vi "PH_TKTDS-30xx.PC Set Channel Position.vi"(0 "i ref in":refnum<vi>, 2 "Channel Name":string(combo)="CH1", 3 "Position (0)":dbl, 5 "error IO":errorcluster) -> (14 "i ref out":refnum<vi>, 19 "error out":errorcluster)   [LabVIEW 2014, in "PH_TKTDS-30xx.lvlib"]
doc: "This case sets the position of the specified channel at the display in display divisions."
uses:
  PH_TKTDS-30xx.lvlib
  instr.lib/TKDS3032-PHELIX/tktds3032-PHELIX - Driver np.lvlib
  PH_Basics/PH_Common/PH_Common.lvlib
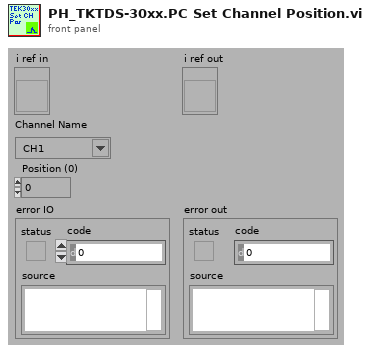
[diagram p1: front panel]
types:
  T1 = typedef "PH_TKTDS-30xx.lvlib/PH_TKTDS-30xx.i attribute.ctl" = cluster{"Default VISA Resource":string, "VISA Resource Name":refnum<visa-resource-name>, "Revision":cluster{"Instrument Driver":string, "Instrument Firmware":string}, "Selftest":cluster{"Result":u32, "Message":string}, "Channels":T2[], "Trigger Configuration":T3, "Acquisition Configuration":T4, "Fetched Waveforms":T5[], "GUI Refs":T6, "GUI Refs Channels":refnum<vi>[], "State":T7, "Error Message":string, "Allow Prdc Loop?":bool}
  T2 = typedef "PH_TKTDS-30xx.lvlib/PH_TKTDS-30xx.Channel Config.ctl" = cluster{"Channel Name":string, "Input Impedance":string, "Max Input Frequency":string, "Vertical Coupling":i32, "Channel Enabled":bool, "Probe Attenuation":dbl, "Vertical Range":dbl, "Vertical Offset":dbl}
  T3 = typedef "PH_TKTDS-30xx.lvlib/PH_TKTDS-30xx.Trigger Config.ctl" = cluster{"Source":string, "Slope":i32, "Level [V]":dbl}
  T4 = typedef "PH_TKTDS-30xx.lvlib/PH_TKTDS-30xx.Acquisition Config.ctl" = cluster{"Time base":dbl, "Record Length":u16, "Start Time":dbl, "Type":i32, "Continuous":bool}
  T5 = typedef "PH_TKTDS-30xx.lvlib/PH_TKTDS-30xx.fetched Waveform.ctl" = cluster{"Source":string, "Actual Points":u32, "Initial X":dbl, "X Increment":dbl, "Waveform Array":dbl[]}
  T6 = typedef "PH_TKTDS-30xx.lvlib/PH_TKTDS-30xx.GUI Refs.ctl" = cluster{"Trigger":refnum<vi>, "Acquisition":refnum<vi>, "Graph":refnum<vi>, "State":refnum<vi>, "Delete":refnum<vi>, "Channel to be positioned":refnum<vi>, "Postion":refnum<vi>, "Display Intensity":refnum<vi>, "VISA Resource":refnum<vi>}
  T7 = typedef "PH_StatusHandler.lvlib/PH_StatusHandler.Status.ctl" = i16
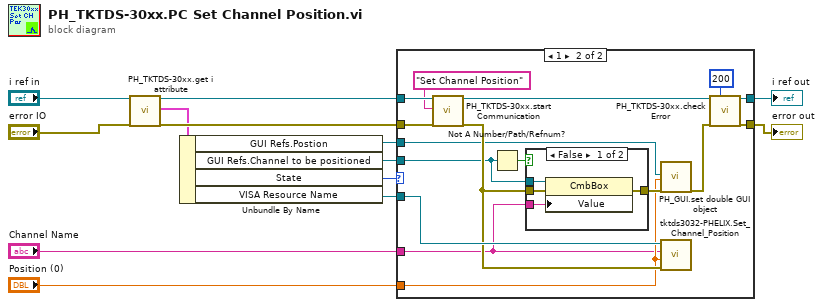
[diagram p0: block diagram]
diagram:
  n1 = call "PH_TKTDS-30xx.get i attribute.vi"("i ref in"="i ref in", "error in (no error)"="error IO") -> ("i ref out"=w8:refnum<vi>, "i attribute"=w10:T1, "error out"=w12:errorcluster)  [unwired: 15 in]
  n2 = Unbundle By Name(w10) -> ("GUI Refs.Postion"=w2:refnum<vi>, "GUI Refs.Channel to be positioned"=w3:refnum<vi>, "State"=w1:T7, "VISA Resource Name"=w11:refnum<visa-resource-name>)
  n3 = case shown="1" w1 {
    tunnel: w8 -> [w15 w31]
    tunnel: w11 -> [_ w30]
    tunnel: [w14 w29] -> w6
    tunnel: w12 -> [w14 w24]
    tunnel: [w15 w28] -> w13
    tunnel: "Channel Name" -> [_ w18]
    tunnel: "Position (0)" -> [_ w19]
    tunnel: w3 -> [_ w16]
    tunnel: w2 -> [_ w20]
    frame Default {
    }
    frame 1 {
      n4 = call "PH_TKTDS-30xx.start Communication.vi"("i ref in"=w31, "Action"="Set Channel Position", "error in"=w24) -> ("i ref out"=w25:refnum<vi>, "error out"=w23:errorcluster)  [unwired: 15 in]
      n5 = Not A Number/Path/Refnum?(number/path/refnum=w16) -> (NaN/Path/Refnum?=w17:bool)
      n6 = case shown="False" w17 {
        tunnel: w23 -> [w35 w36]
        tunnel: [w34 w36] -> w22
        tunnel: w16 -> [w33 _]
        tunnel: w18 -> [w32 _]
        frame False {
          n7 = property class="CmbBox"(reference=w33, error in=w35, "Value"=w32) -> (error out=w34:errorcluster)  [unwired: 1 out]
        }
        frame True {
        }
      }
      n8 = call "PH_GUI.set double GUI object.vi"("GUI object Ref"=w20, "value"=w19, "error in (no error)"=w22) -> ("error out"=w21:errorcluster)  [unwired: 16 in]
      n9 = call "tktds3032-PHELIX.Set_Channel_Position.vi"("error in (no error)"=w23, "Position (0)"=w19, "Channel Name (\"CH1\")"=w18, "VISA Resource Name"=w30) -> ()  [unwired: 6 in, 2 out]
      n10 = call "PH_TKTDS-30xx.check Error.vi"("i ref in"=w25, "Waiting Time [ms]"=u32 200, "error in"=w21) -> ("i ref out"=w28:refnum<vi>, "error out"=w29:errorcluster)  [unwired: 15 in]
    }
  }
  "i ref out" <- w13
  "error out" <- w6
